vi "Get Custom Device Properties.vi"   [LabVIEW 2013, in "J1939 System Definition API.lvlib"]
uses:
  J1939 System Definition API.lvlib
  J1939 System Definition API Support.lvlib
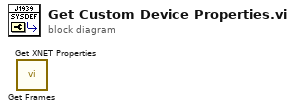
[diagram p0: block diagram]
diagram:
  n1 = call "Get Frames.vi"() -> ()  [unwired: 9 in, 3 out]
  n2 = call "Get XNET Properties.vi"() -> ()  [unwired: 9 in, 3 out]
